vi "MUSIC (Host).vi"() -> ()   [LabVIEW 2020]
doc: "This template is for the Simple NI-USRP Streaming design, a design that shows the basics of streaming data from an NI 294x/295x device. Refer to the block diagram for more information about how to use this template."
uses:
  SubVIs/Start Trigger.ctl
  <vilib>/userdefined/Silver/nirio_resource_slv.ctl
  <vilib>/Utility/error.llb/DialogType.ctl
  SubVIs/Streaming Xvcr FPGA Ref.ctl
  <vilib>/Utility/error.llb/Error Cluster From Error Code.vi
  <vilib>/rvi/errors/niLvFpgaAdjustHostInterfaceError.vi
  <vilib>/rvi/interface/nirviReadWriteControl/nirviReadWriteControl.xnode
  <vilib>/rvi/interface/Simulation/niFpgaSimulationCallBeginRW.vi
  NiFpgaLv.dll
panel:
  in  "servo angle":i8
  in  "make turn":bool
  in  "VISA resource name":refnum<visa-resource-name>
  out "signal power":dbl
  out "noise power":dbl
  out "?":cluster{i32[], "CSI abs":dbl[]}[](graph)
  out "acquiring":bool caption="Acquiring"
  in  "rx.stop":bool
  out "?":bool
  out "?":dbl
  out "?":u32
  out "SNR (dB)":dbl(knob) scale=-10.0..20.0
  in  "SNR threshold (dB)":dbl(slide)=12.121212121212121 scale=-1.0..20.0
  out "SNRs in FIFO":u32(slide) scale=0.0..100.0
  in  "?":enum32{""}(tab)
  out "?":cluster{dbl[], dbl[]}(graph)
  out "AoA":dbl(knob) scale=-90.0..90.0
  out "?":dbl
  out "CSI in FIFO":u32(slide) scale=0.0..24200.0
  out "?":u32
  in  "?":enum32{""}(tab)
  out "?":cluster{dbl[], dbl[]}(graph)
  out "AoA":dbl(knob) scale=-90.0..90.0
  out "?":dbl
  out "samples in FIFO":u32(slide) scale=0.0..100000.0
  out "?":u32
  in  "send before CFO":bool
  in  "?":enum32{""}(tab)
  in  "phases 2":T1 {"channel 1" scale=0.0..1.0; "channel 2" scale=0.0..1.0; "channel 3" scale=0.0..1.0; "channel 4" scale=0.0..1.0}
  in  "phases":T1={"channel 1"=0.0, "channel 2"=0.2256, "channel 3"=0.7026, "channel 4"=0.4525}
  in  "?":bool
  in  "before CFO compensation":bool
  in  "rx config":T3={"transfer mode"=enum."Finite", "sample rate"=80000000.0, "number of samples"=8192, "start trigger"=enum."Immediate", "daughterboard 0 config"={"rf enable 0"=TRUE, "rf config 0"={"antenna"="RX1", "frequency"=2475000000.0, "gain"=60.0}, "rf enable 1"=TRUE, "rf config 1"={"antenna"="RX2", "frequency"=2475000000.0, "gain"=60.0}, "lo configuration"=enum."Import"}, "daughterboard 1 config"={"rf enable 2"=TRUE, "rf config 2"={"antenna"="RX1", "frequency"=2475000000.0, "gain"=60.0}, "rf enable 3"=TRUE, "rf config 3"={"antenna"="RX2", "frequency"=2475000000.0, "gain"=60.0}, "lo configuration"=enum."Shared and Export"}} {"daughterboard 1 config"."rf config 3"."gain" format="%#.1f"; "daughterboard 1 config"."rf config 3"."frequency" format="%#.3pHz"; "daughterboard 1 config"."rf config 2"."gain" format="%#.1f"; "daughterboard 1 config"."rf config 2"."frequency" format="%#.3pHz"; "daughterboard 0 config"."rf config 1"."gain" format="%#.1f"; "daughterboard 0 config"."rf config 1"."frequency" format="%#.3pHz"; "daughterboard 0 config"."rf config 0"."gain" format="%#.1f"; "daughterboard 0 config"."rf config 0"."frequency" format="%#.3pHz"; "sample rate" format="%#.3pS/s"}
  in  "indicator tab":T4(tab)
  in  "configuration":T5={"primary channel selector"=0.25, "last OFDM symbol index"=10, "switch format detection states"=FALSE, "format"=enum."VHT", "bandwidth"=enum."80MHz"}
  in  "for shift":T6(ring)=enum."10MHz"
  in  "for filter":enum16{"20MHz", "40MHz"}(ring)
  out "subcar ind":fxp<+/-,9,9>
  out "channel estimate valid":bool
  out "channel estimate":T7
  out "pack num":u32
  out "was pack detected true?":bool
  out "was packet start true?":bool
  out "packet detected":bool
  out "packet start":bool
  in  "USRP RIO device":T8="RIO0" caption="USRP RIO Device"
  in  "reference frequency source":string(combo)="Internal" caption="Reference Frequency Source"
  out "sample out":T9
  out "sample out valid":bool
  in  "use statuc freq shift":bool
  out "compensated CFO":fxp<+/-,48,0>
  out "rx.coerced config":T10 {"channel 3"."sample rate" format="%#.3pS/s"; "channel 3"."gain" format="%#_1f"; "channel 3"."if2 lo" format="%#.3pHz"; "channel 3"."if1 lo" format="%#.3pHz"; "channel 3"."frequency" format="%#.3pHz"; "channel 2"."sample rate" format="%#.3pS/s"; "channel 2"."gain" format="%#_1f"; "channel 2"."if2 lo" format="%#.3pHz"; "channel 2"."if1 lo" format="%#.3pHz"; "channel 2"."frequency" format="%#.3pHz"; "channel 1"."sample rate" format="%#.3pS/s"; "channel 1"."gain" format="%#_1f"; "channel 1"."if2 lo" format="%#.3pHz"; "channel 1"."if1 lo" format="%#.3pHz"; "channel 1"."frequency" format="%#.3pHz"; "channel 0"."sample rate" format="%#.3pS/s"; "channel 0"."gain" format="%#_1f"; "channel 0"."if2 lo" format="%#.3pHz"; "channel 0"."if1 lo" format="%#.3pHz"; "channel 0"."frequency" format="%#.3pHz"}
  in  "packet number":u32=30
  out "packet number in buf":u32=30
  out "packets in buf (%)":dbl(slide)=1000.0 scale=0.0..1.0
  out "csi string buffer":string
  out "samples string buffer":string
  in  "?":bool
  in  "experiment name":string="test"
  out "Done":bool=TRUE
  # "MUSIC Localization"
  # "Orion"
  # "ArrayTrack"
  # "signal *= exp(i*2*pi*phases) / 4\nNeed to recompute power"
  # "from RF"
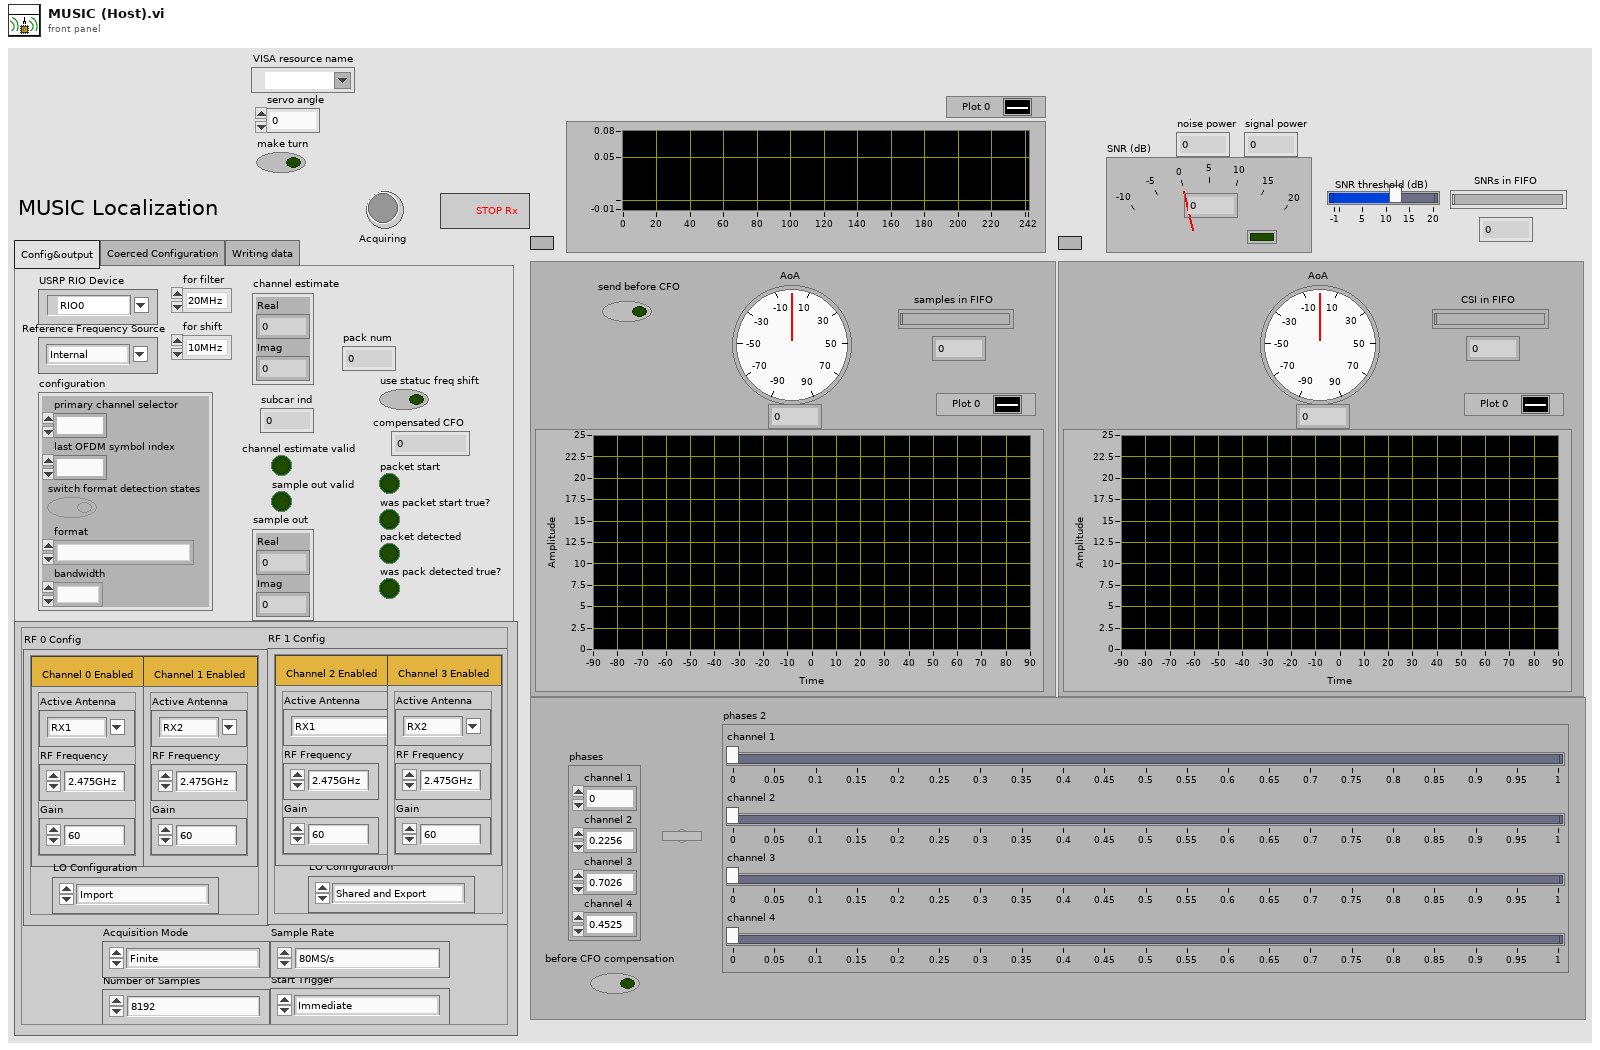
[diagram p1: front panel]
types:
  T1 = cluster{"channel 1":dbl, "channel 2":dbl, "channel 3":dbl, "channel 4":dbl}
  T2 = typedef "Start Trigger.ctl" = enum8{"Software", "Digital Edge", "Rx Start Trigger", "Tx Start Trigger", "Immediate", "Future Time Event"}
  T3 = cluster{"transfer mode":enum16{"Finite", "Continuous"}, "sample rate":dbl, "number of samples":u32, "start trigger":T2, "daughterboard 0 config":cluster{"rf enable 0":bool, "rf config 0":cluster{"antenna":string, "frequency":dbl, "gain":dbl}, "rf enable 1":bool, "rf config 1":cluster{"antenna":string, "frequency":dbl, "gain":dbl}, "lo configuration":enum16{"Independent", "Import", "Shared and Export", "Reimport", "Shared"}}, "daughterboard 1 config":cluster{"rf enable 2":bool, "rf config 2":cluster{"antenna":string, "frequency":dbl, "gain":dbl}, "rf enable 3":bool, "rf config 3":cluster{"antenna":string, "frequency":dbl, "gain":dbl}, "lo configuration":enum16{"Independent", "Import", "Shared and Export", "Reimport", "Shared"}}}
  T4 = enum32{"Config&output", "Coerced Configuration", "Writing data"}
  T5 = cluster{"primary channel selector":fxp<+,2,0>, "last OFDM symbol index":u16, "switch format detection states":bool, "format":enum16{"NON_HT_OFDM", "VHT", "NON_HT_DUP_OFDM"}, "bandwidth":enum16{"20MHz", "40MHz", "80MHz"}}
  T6 = enum16{"-30MHz", "-20MHz", "-10MHz", "0MHz", "10MHz", "20MHz", "30MHz"}
  T7 = cluster{"Real":fxp<+/-,25,4>, "Imag":fxp<+/-,25,4>}
  T8 = typedef "nirio_resource_slv.ctl" = tag
  T9 = cluster{"Real":fxp<+/-,16,3>, "Imag":fxp<+/-,16,3>}
  T10 = cluster{"channel 0":cluster{"frequency":dbl, "if1 lo":dbl, "if2 lo":dbl, "gain":dbl, "sample rate":dbl}[], "channel 1":cluster{"frequency":dbl, "if1 lo":dbl, "if2 lo":dbl, "gain":dbl, "sample rate":dbl}[], "channel 2":cluster{"frequency":dbl, "if1 lo":dbl, "if2 lo":dbl, "gain":dbl, "sample rate":dbl}[], "channel 3":cluster{"frequency":dbl, "if1 lo":dbl, "if2 lo":dbl, "gain":dbl, "sample rate":dbl}[], "device id":i32}
  T11 = typedef "DialogType.ctl" = u16
  T12 = typedef "Rx Channels.ctl" = cluster{"rx config":cluster{"channel configuration":cluster{"channel enable":bool, "channel configuration":cluster{"antenna":string, "frequency":dbl, "lo frequency":dbl, "level":dbl}}[], "transfer mode":enum16{"Finite", "Continuous"}, "sample rate":dbl, "number of samples":u32, "start trigger":T2}, "reference frequency source":string, "rx.data sink":enum16{"SFP Port 0", "SFP Port 1", "Host"}, "rx.enabled channels":string[], "vertical range":dbl[], "rx.coerced configurations":cluster{"coerced frequencies":dbl[], "coerced lo frequencies":dbl[], "coerced levels":dbl[], "coerced sample rates":dbl[]}}
  T13 = typedef "niUsrpRio Config v1 Host.lvlib/niUsrpRio Session.ctl" = cluster{"FPGA Interface":refnum<k20>, "RIO Interface Number":u32, "Data Clock Rate":u32, "FPGA Data Clock Rate":u32, "Global Settings Register Bus":T14, "Radio 0 Settings Register Bus":T14, "Radio 1 Settings Register Bus":T14, "Radio Settings Bus Semaphore":T15, "DB Queues":T16[], "Characterization Data Valid?":bool, "EEPROM Header":T17, "Device Data Header":T18, "EEPROM Characterization Header":T19, "Characterization Data":T20[], "FPGA Current Version":u32, "FPGA Oldest Compatible Version":u32, "Fixed Logic Current Version":u32, "Fixed Logic Oldest Compatible Version":u32, "FPGA Radio Settings Bus Current Version":u32, "FPGA Radio Settings Bus Oldest Compatible Version":u32, "FPGA Board Config Current Version":u32, "FPGA Board Config Oldest Compatible Version":u32, "Daughterboard Clock Rate":u32, "daughterboard configuration session handles":u64[]}
  T14 = typedef "niInstr Register Bus v0 Host.lvlib/Register Bus Session.ctl" = refnum<queue>
  T15 = typedef "Semaphore RefNum" = refnum<k1>
  T16 = typedef "niUsrpRio Config v1 Host.lvlib/DB Queue Reference.ctl" = refnum<queue>
  T17 = typedef "niUsrpRio Config v1 Host.lvlib/EEPROM Header.ctl" = cluster{"Checksum":u32, "Product Code":u16, "Hardware Current Version":u16, "Hardware Oldest Compatible Version":u16, "EEPROM Map Current Version":u16, "EEPROM Map Oldest Compatible Version":u16, "User Password":string, "Pointer to Factory Header":u32, "Pointer to User Header":u32, "Recommended Interval":u16, "Number of Reserved Bytes":i32, "Number of Daughterboards":u8, "Daughterboard IDs":u16[], "Daughterboard Serial Numbers":string[]}
  T18 = typedef "niUsrpRio Config v1 Host.lvlib/EEPROM Device Data Header.ctl" = cluster{"Checksum":u32, "Number of Channels":u8, "Number of Gain Settings":u16[], "Pointer to Characterization Data":u32[], "Number of Reserved Bytes":i32, "Number of Frequencies":u16[]}
  T19 = typedef "niUsrpRio Config v1 Host.lvlib/EEPROM Characterization Header.ctl" = cluster{"Checksum":u32, "Date":timestamp, "Temperature":sgl, "Misc. Info":string, "Pointer to Device Data Header":u32, "Number of Reserved Bytes":i32}
  T20 = typedef "niUsrpRio Config v1 Host.lvlib/Characterization Data.ctl" = cluster{"Gains[dB]":dbl[], "Frequencies [Hz]":dbl[], "IQ Imbalance Table":T21[], "Measured Gains[dB]":dbl[][]}
  T21 = typedef "niUsrpRio Config v1 Host.lvlib/IQ Imbalance.ctl" = cluster{"Gain Imbalance [linear]":dbl, "Phase Imbalance [radians]":dbl, "Offset":cdb}
  T22 = cluster{"coerced frequencies":dbl[], "coerced if1 frequencies":dbl[], "coerced if2 frequencies":dbl[], "coerced gain":dbl[], "coerced sample rates":dbl[]}
  T23 = typedef "Streaming Xvcr FPGA Ref.ctl" = refnum<k20>
  T24 = cluster{"channel 1 ":cluster{"Real":fxp<+/-,16,3>, "Imag":fxp<+/-,16,3>}, "channel  2":cluster{"Real":fxp<+/-,16,3>, "Imag":fxp<+/-,16,3>}, "channel  3":cluster{"Real":fxp<+/-,16,3>, "Imag":fxp<+/-,16,3>}, "channel  4":cluster{"Real":fxp<+/-,16,3>, "Imag":fxp<+/-,16,3>}}
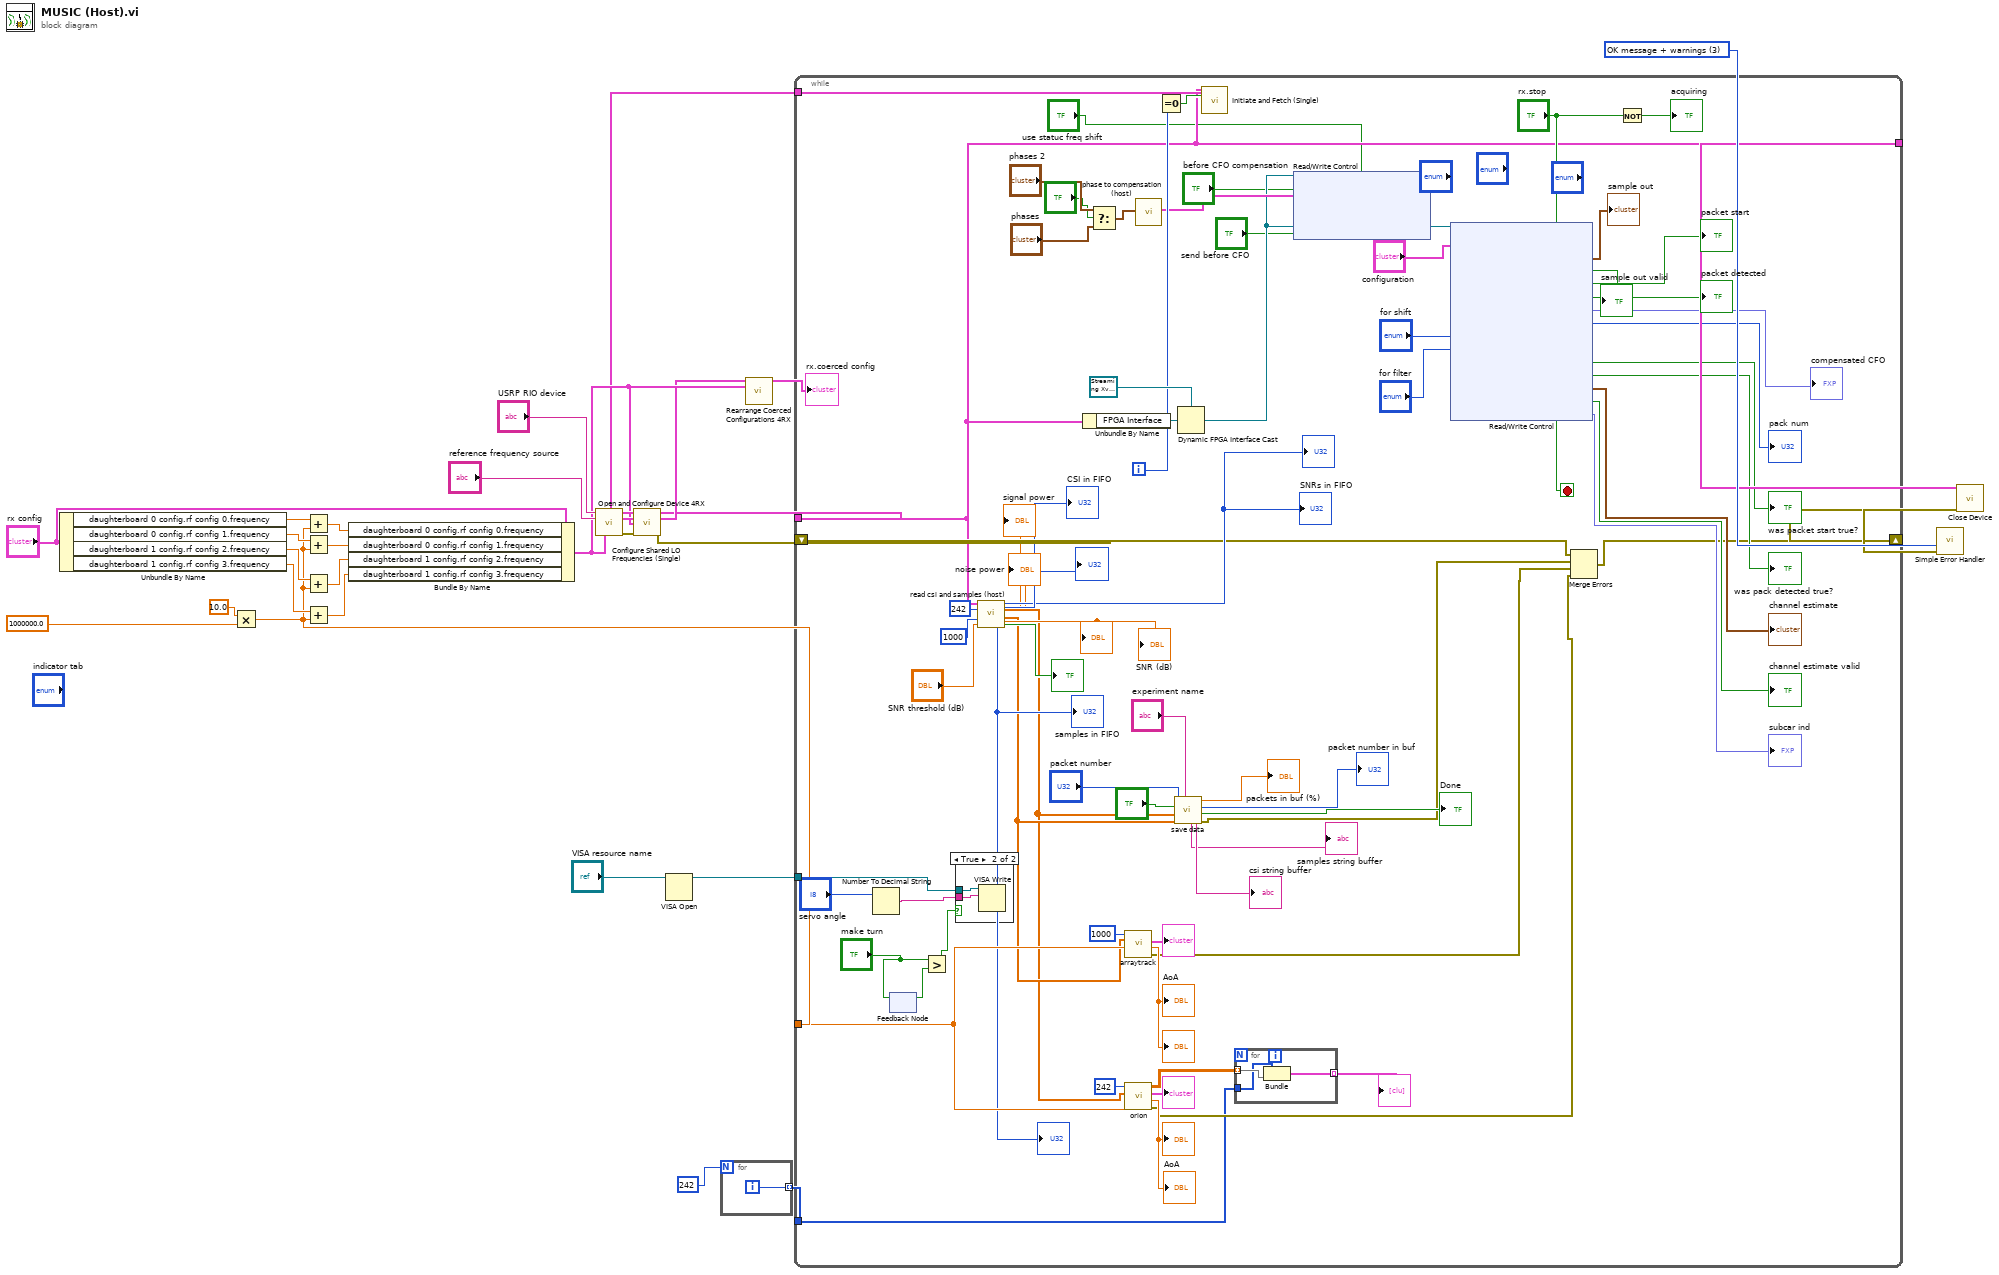
[diagram p0: block diagram]
diagram:
  w31 = T11 3 items=["no dialog", "OK message", "continue or stop message", "OK message + warnings", "continue/stop + warnings"] ("type of dialog (OK msg:1)")
  n1 = Unbundle By Name("rx config") -> ("daughterboard 0 config.rf config 0.frequency"=w17:dbl, "daughterboard 0 config.rf config 1.frequency"=w16:dbl, "daughterboard 1 config.rf config 2.frequency"=w15:dbl, "daughterboard 1 config.rf config 3.frequency"=w14:dbl)
  n2 = Multiply(x=10.0 ("daughterboard 1 config.rf config 3.frequency"), y=1000000.0) -> (x*y=w9:dbl)
  n3 = Add(x=w17, y=w9) -> (x+y=w21:dbl)
  n4 = Add(x=w16, y=w9) -> (x+y=w18:dbl)
  n5 = Add(x=w15, y=w9) -> (x+y=w19:dbl)
  n6 = Add(x=w14, y=w9) -> (x+y=w20:dbl)
  n7 = Bundle By Name(cluster="rx config", "daughterboard 0 config.rf config 0.frequency"=w21, "daughterboard 0 config.rf config 1.frequency"=w18, "daughterboard 1 config.rf config 2.frequency"=w19, "daughterboard 1 config.rf config 3.frequency"=w20) -> (w12:T3)
  n8 = call "Open and Configure Device 4RX.vi"("USRP RIO Device"="USRP RIO device", "reference frequency source"="reference frequency source", "rx config"=w12) -> ("rx channels"=w8:T12, "niUsrpRio Session (out)"=w25:T13, "rx.coerced configurations"=w22:T22, "error out"=w23:errorcluster)  [unwired: 9 in]
  n9 = call "Configure Shared LO Frequencies (Single).vi"("niUsrpRio Session"=w25, "rx.coerced config"=w22, "rx config"=w12, "error in"=w23) -> ("niUsrpRio Session (out)"=w6:T13, "rx.coerced config out"=w7:T22, "error out"=w24:errorcluster)  [unwired: 9 in]
  n10 = VISA Open(VISA resource name="VISA resource name") -> (VISA resource name=w1:refnum<visa-resource-name>)  [unwired: 4 in, 1 out]
  n11 = for {
    N: u32 242 ("samples num") -> [_]
    tunnel: [w32] -> w3 mode=indexing
    i -> [w32]
  }
  n12 = call "Rearrange Coerced Configurations 4RX.vi"("rx.coerced configurations"=w7, "rx config"=w12) -> ("coerced configurations"=→"rx.coerced config":T10)  [unwired: 13 in]
  n13 = while {
    tunnel: w6 -> [w74]
    tunnel: [w74] -> w26
    shift-right: [w52] -> w27
    shift-left: w24 -> [w53]
    tunnel: w9 -> [w72]
    tunnel: w8 -> [w88]
    tunnel: w3 -> [w46]
    tunnel: w1 -> [w42]
    i -> [w90]
    stop <- "rx.stop" stop-if-true
    # "Acquire and Fetch a waveform"
    n14 = Number To Decimal String(number="servo angle") -> (decimal integer string=w38:string)  [unwired: 1 in]
    n15 = feedback-in #1("make turn") -> ()
    n16 = feedback #1() -> (w39:bool)  [unwired: 1 in]
    n17 = Greater?(x="make turn", y=w39) -> (0:w40:bool)
    n18 = case shown="True" w40 {
      tunnel: w42 -> [_ w106]
      tunnel: w38 -> [_ w105]
      frame False {
      }
      frame True {
        n19 = VISA Write(VISA resource name=w106, write buffer=w105) -> ()  [unwired: 1 in, 3 out]
      }
    }
    n20 = call "read csi and samples (host).vi"("input cluster"=w74, "csi num"=u32 242, "samples num"=u32 1000, "SNR threshold"="SNR threshold (dB)") -> ("signal power"=→"signal power":dbl, "noise power"=→"noise power":dbl, "CSI Remaining"=→"CSI in FIFO" →"?":u32, "Power measurements Remaining"=→"SNRs in FIFO" →"?":u32, "csi"=w48:cdb[], "samples"=w61:cdb[], "SNR"=→"SNR (dB)" →"?":dbl, "samples remaining"=→"samples in FIFO" →"?":u32, "packet valid"=→"?":bool)  [unwired: 3 in]
    n21 = Unbundle By Name(w74) -> ("FPGA Interface"=w83:refnum<k20>)
    n22 = Select(t="phases 2", s="?", f="phases") -> (s? t:f=w85:T1)
    n23 = call "arraytrack.vi"("freq"=w72, "samples"=w61, "samples num"=u32 1000) -> ("error out"=w50:errorcluster, "max"=→"AoA" →"?":dbl, "spectrum"=→"?":cluster{dbl[], dbl[]})  [unwired: 6 in]
    n24 = call "orion.vi"("freq"=w72, "csi"=w48, "csi num"=u32 242 ("samples num")) -> ("error out"=w49:errorcluster, "max"=→"?" →"AoA":dbl, "spectrum"=→"?":cluster{dbl[], dbl[]}, "CSI abs"=w47:dbl[][])  [unwired: 5 in]
    n25 = call "phase to compensation (host).vi"("phases"=w85) -> ("for comp"=w87:T24)  [unwired: 10 in]
    n26 = Equal To 0?(x=w90) -> (x = 0?=w89:bool)
    n27 = call "save data.vi"("experiment name"="experiment name", "samples"=w61, "csi"=w48, 10:"?", "packet number"="packet number") -> ("error out"=w51:errorcluster, "Done"=→"Done":bool, "packet number in buf"=→"packet number in buf":u32, "packets in buf (%)"=→"packets in buf (%)":dbl, "samples string buffer"=→"samples string buffer":string, "csi string buffer"=→"csi string buffer":string)  [unwired: 1 in]
    n28 = Dynamic FPGA Interface Cast(Session In=T23 refnum ("Type"), Type=w83) -> (Session Out=w82:T23)
    n29 = call "Initiate and Fetch (Single).vi"("niUsrpRio Session"=w74, "rx channels"=w88, "first iteration"=w89) -> ()  [unwired: 10 in, 3 out]
    n30 = for {
      tunnel: w47 -> [w108] mode=indexing
      tunnel: w46 -> [w107]
      tunnel: [w109] -> w45 mode=indexing
      n31 = Bundle(w107, "CSI abs"=w108) -> (w109:cluster{i32[], "CSI abs":dbl[]})  [unwired: 1 in]
    }
    "?" <- w45
    n32 = xnode "Read/Write Control"("FPGA VI Reference In"=w82, "compensation"=w87, "use static frequency shift"="use statuc freq shift", "before CFO compensation"="before CFO compensation", "save before CFO"="send before CFO") -> ()  [unwired: 1 in, 2 out]
    n33 = xnode "Read/Write Control"("FPGA VI Reference In"=w82, "configuration"="configuration", "for shift"="for shift", "for filter"="for filter") -> ("sample out"=→"sample out":T9, "sample out valid"=→"sample out valid":bool, "packet start"=→"packet start":bool, "packet detected"=→"packet detected":bool, "compensated CFO"=→"compensated CFO":fxp<+/-,48,0>, "packet start number"=→"pack num":u32, "was packet start true?"=→"was packet start true?":bool, "was packet detected true? 2"=→"was pack detected true?":bool, "channel estimate"=→"channel estimate":T7, "channel estimate valid"=→"channel estimate valid":bool, "subcarrier index"=→"subcar ind":fxp<+/-,9,9>)  [unwired: 1 in, 2 out]
    n34 = Merge Errors(w53, w51, w50, w49) -> (w52:errorcluster)
    n35 = Not(x="rx.stop") -> (.not. x?=→"acquiring":bool)
  }
  n36 = call "Close Device.vi"("niUsrpRio Session"=w26, "error in"=w27) -> ("error out"=w30:errorcluster)  [unwired: 13 in]
  n37 = call <vilib>:"Simple Error Handler.vi"("type of dialog (OK msg:1)"=w31, "error in (no error)"=w30) -> ()  [unwired: 3 in, 5 out]
